vi "Fly.vi"(10 "Sol_RaiseDrop":T1, 11 "Joy_R Buttons":bool[](array[boolean])) -> (3 "Flywheel output":dbl)   [LabVIEW 2017]
uses:
  <vilib>/Rock Robotics/WPI/Solenoid/WPI_SolenoidValue.ctl
  TypeDefs/joybuttons.ctl
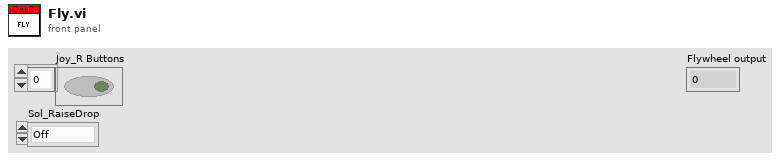
[diagram p1: front panel]
types:
  T1 = typedef "WPI_SolenoidValue.ctl" = enum16{"Off", "On", "Forward", "Reverse"}
  T2 = typedef "joybuttons.ctl" = enum16{"Trigger", "Thumb", "Top3", "Top4", "Top5", "Top6", "Bottom7", "Bottom8", "Bottom9", "Bottom10", "Bottom11", "Bottom12", ""}
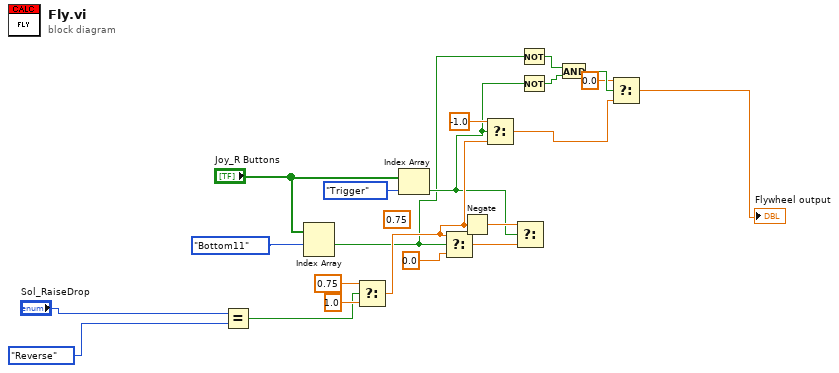
[diagram p0: block diagram]
diagram:
  (unwired) 0.75
  n1 = Equal?(x="Sol_RaiseDrop", y=WPI_SolenoidValue."Reverse" ("Previous Sol_RaiseDrop 2")) -> (x = y?=w11:bool)
  n2 = Index Array(array="Joy_R Buttons", index #1=joybuttons."Bottom11" ("Enum")) -> (element #1=w5:bool)  [unwired: 1 in, 1 out]
  n3 = Select(t=0.75, s=w11, f=1.0) -> (s? t:f=w9:dbl)
  n4 = Index Array(array="Joy_R Buttons", index=joybuttons."Trigger" ("Enum")) -> (element=w6:bool)
  n5 = Select(t=w9, s=w5, f=0.0) -> (s? t:f=w19:dbl)
  n6 = Negate(x=w9) -> (-x=w18:dbl)
  n7 = Select(t=-1.0, s=w6, f=w9) -> (s? t:f=w3:dbl)
  n8 = Select(t=w18, s=w6, f=w19) -> ()  [unwired: 1 out]
  n9 = Not(x=w5) -> (.not. x?=w8:bool)
  n10 = Not(x=w6) -> (.not. x?=w7:bool)
  n11 = And(x=w8, y=w7) -> (x .and. y?=w4:bool)
  n12 = Select(t=0.0, s=w4, f=w3) -> (s? t:f=→"Flywheel output":dbl)
